vi "Cool vision code.vi"(11 "Image":T1) -> (1 "Original Image":T1(plugin-control), 2 "Distance (ft)":dbl, 3 "Mask":T1(plugin-control))   [LabVIEW 2019]
uses:
  Support/Camera Types.ctl
  <vilib>/vision/Image Controls.llb/IMAQ Image.ctl
  <vilib>/vision/NI_Vision_Development_Module.lvlib
panel:
  out "Disqualified":i32=13
  out "Results":T2(array[cluster])=[{"diameter points"={"first point"={"x"=213.0, "y"=163.0}, "projected point"={"x"=293.0, "y"=194.0}}, "Normalized Center"={"x"=0.58125, "y"=0.48750000000000004}, "Overall Score"=61.175669724085026, "Area Score"=96.13589211618256, "Moment Score"=62.73202614698161, "Aspect Score"=24.659090909090907, "Distance (ft)"=4.347709612348454, "Upper Goal"=FALSE}, {"diameter points"={"first point"={"x"=243.0, "y"=142.0}, "projected point"={"x"=266.0, "y"=171.0}}, "Normalized Center"={"x"=0.5906250000000002, "y"=0.3041666666666667}, "Overall Score"=74.56623386292142, "Area Score"=82.18546637744035, "Moment Score"=61.2760810611263, "Aspect Score"=80.23715415019763, "Distance (ft)"=15.122468216864188, "Upper Goal"=FALSE}] {"Normalized Center"."x" format="%#_2g"; "Normalized Center"."y" format="%#_2g"; "Overall Score" format="%#_2g"; "Distance (ft)" format="%#_3g"; "Area Score" format="%#_2g"; "Moment Score" format="%#_2g"; "Aspect Score" format="%#_2g"}
  in  "Size Limit %":dbl=0.04 min=0.0 max=100.0 step=0.01 format="%#_13g"
  in  "Color Mode":u16(ring)=2 items=["RGB", "HSL", "HSV", "HSI"]
  in  "Particle Count":i32=5
  in  "Score Threshold %":dbl=75.0
  in  "Std Devs for Calibration":cluster{"H":dbl, "S":dbl, "V":dbl}={"H"=4.0, "S"=8.0, "V"=8.0}
  in  "Camera Type (for distance)":T3=enum."MS HD3000 square"
  in  "Annotate":bool=TRUE
  out "Qualified":i32=5
  in  "LED Color Range":T4={"Hue"={14.360681298918061, 47.91090746924753}, "Sat"={75.89285714285714, 255.0}, "Val"={97.14285714285714, 251.32874298095703}} {"Hue" scale=0.0..255.0 scale format="%#_3g"}
  # "Limits"
  # "Particle Results"
  # "Good target"
  # "Disqualified"
  # "Distance (ft)"
  # "Scores"
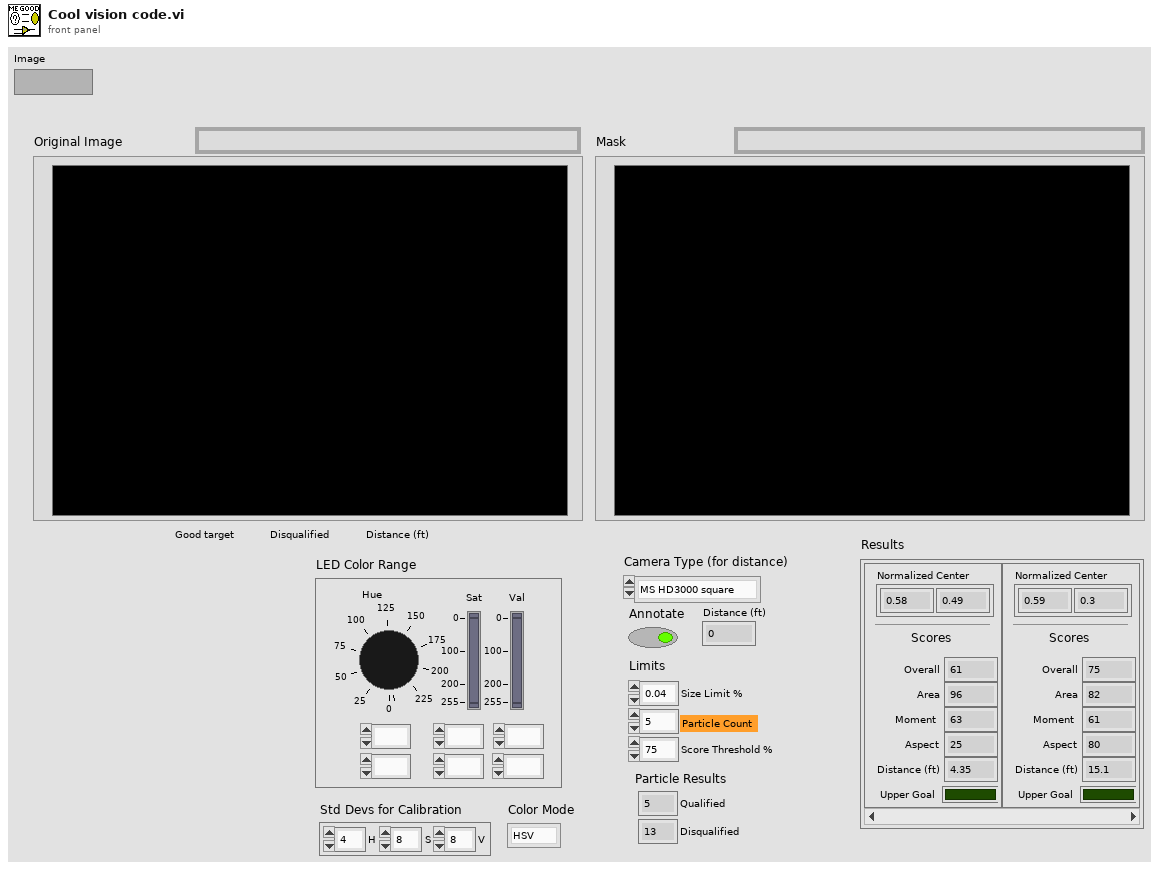
[diagram p1: front panel]
types:
  T1 = typedef "IMAQ Image.ctl" = refnum<image>
  T2 = cluster{"diameter points":cluster{"first point":cluster{"x":dbl, "y":dbl}, "projected point":cluster{"x":dbl, "y":dbl}}, "Normalized Center":cluster{"x":dbl, "y":dbl}, "Overall Score":dbl, "Area Score":dbl, "Moment Score":dbl, "Aspect Score":dbl, "Distance (ft)":dbl, "Upper Goal":bool}[]
  T3 = typedef "Camera Types.ctl" = enum16{"206", "1011", "1013", "MS HD3000 square", "MS HD3000 640x480"}
  T4 = cluster{"Hue":cluster{dbl, dbl}, "Sat":cluster{dbl, dbl}, "Val":cluster{dbl, dbl}}
  T5 = typedef "Particle Parameters" = i32
  T6 = typedef "Image Type" = u32
  T7 = enum32{"AutoM", "Close", "Dilate", "Erode", "Gradient", "Gradient out", "Gradient in", "Hit miss", "Open", "PClose", "POpen", "Thick", "Thin"}
  T8 = cluster{cluster{dbl, dbl}, cluster{dbl, dbl}, cluster{dbl, dbl}}
  T9 = cluster{"remainder":i32, "size":bool, "count":bool}
  T10 = typedef "Target Fields.ctl" = cluster{"diameter points":cluster{"first point":cluster{"x":dbl, "y":dbl}, "projected point":cluster{"x":dbl, "y":dbl}}, "normalized center":cluster{"x":dbl, "y":dbl}, "Overall Score":dbl, "Area Score":dbl, "Moment Score":dbl, "Aspect Score":dbl, "Distance (ft)":dbl, "Upper Goal":bool}
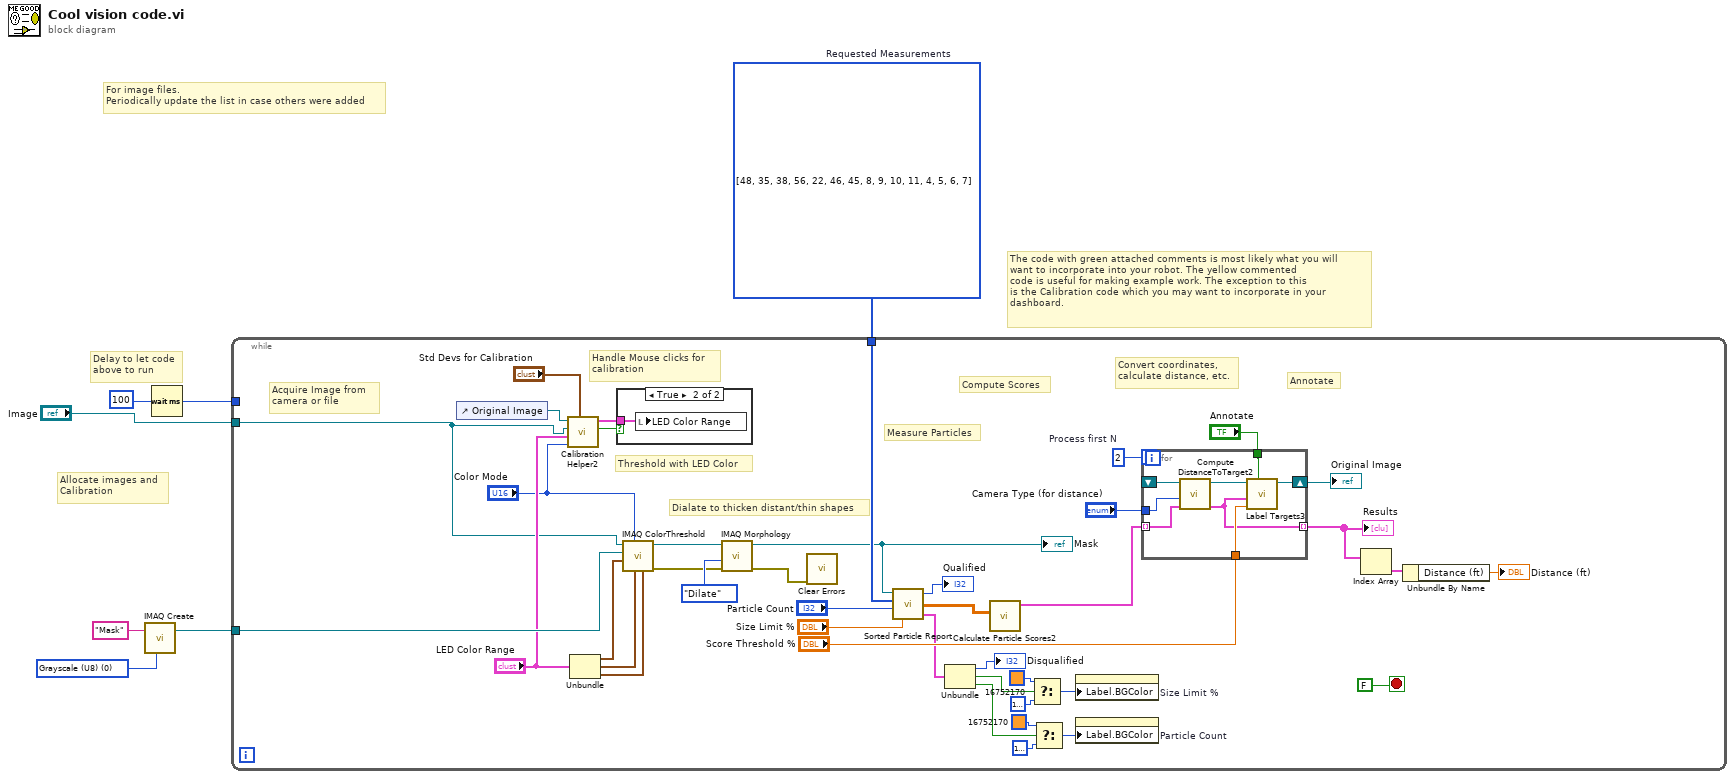
[diagram p0: block diagram]
diagram:
  w4 = T5[] [48, 35, 38, 56, 22, 46, 45, 8, 9, 10, 11, 4, 5, 6, 7] items=["Center of Mass X", "Center of Mass Y", "First Pixel X", "First Pixel Y", "Bounding Rect Left", "Bounding Rect Top", "Bounding Rect Right", "Bounding Rect Bottom", "Max Feret Diameter Start X", "Max Feret Diameter Start Y", "Max Feret Diameter End X", "Max Feret Diameter End Y", "Max Horiz. Segment Length Left", "Max Horiz. Segment Length Right", "Max Horiz. Segment Length Row", "-", "Bounding Rect Width", "Bounding Rect Height", "Bounding Rect Diagonal", "Perimeter", "Convex Hull Perimeter", "Holes' Perimeter", "Max Feret Diameter", "Equivalent Ellipse Major Axis", "Equivalent Ellipse Minor Axis", "Equivalent Ellipse Minor Axis (Feret)", "Equivalent Rect Long Side", "Equivalent Rect Short Side", "Equivalent Rect Diagonal", "Equivalent Rect Short Side (Feret)", "Average Horiz. Segment Length", "Average Vert. Segment Length", "Hydraulic Radius", "Waddel Disk Diameter", "-", "Area", "Holes' Area", "Particle & Holes' Area", "Convex Hull Area", "Image Area", "-", "Number of Holes", "Number of Horiz. Segments", "Number of Vert. Segments", "-", "Orientation", "Max Feret Diameter Orientation", "-", "% Area/Image Area", "% Area/(Particle & Holes' Area)", "Ratio of Equivalent Ellipse Axes", "Ratio of Equivalent Rect Sides", "-", "Elongation Factor", "Compactness Factor", "Heywood Circularity Factor", "Type Factor", "-", "Sum X", "Sum Y", "Sum XX", "Sum XY", "Sum YY", "Sum XXX", "Sum XXY", "Sum XYY", "Sum YYY", "-", "Moment of Inertia XX", "Moment of Inertia XY", "Moment of Inertia YY", "Moment of Inertia XXX", "Moment of Inertia XXY", "Moment of Inertia XYY", "Moment of Inertia YYY", "Norm. Moment of Inertia XX", "Norm. Moment of Inertia XY", "Norm. Moment of Inertia YY", "Norm. Moment of Inertia XXX", "Norm. Moment of Inertia XXY", "Norm. Moment of Inertia XYY", "Norm. Moment of Inertia YYY", "Hu Moment 1", "Hu Moment 2", "Hu Moment 3", "Hu Moment 4", "Hu Moment 5", "Hu Moment 6", "Hu Moment 7"]  # Requested Measurements
  w7 = T6 0 items=["Grayscale (U8)", "Grayscale (I16)", "Grayscale (SGL)", "Complex (CSG)", "RGB (U32)", "HSL (U32)", "RGB (U64)", "Grayscale (U16)"] ("Image Type")
  # "Delay to let code\nabove to run"
  # "The code with green attached comments is most likely what you will\nwant to incorporate into your robot. The yellow commented\ncode is useful for making example work. The exception to this\nis the Calibration code which you may want to incorporate in your\ndashboard."
  # "For image files.\nPeriodically update the list in case others were added"
  # "Allocate images and\nCalibration"
  n1 = call "IMAQ Create"("Image Name"="Mask", "Image Type"=w7) -> ("New Image"=w5:T1)  [unwired: 2 in, 2 out]
  n2 = Wait (ms)(milliseconds to wait=u32 100) -> (millisecond timer value=w3:u32)
  n3 = while {
    tunnel: w5 -> [w47]
    tunnel: w4 -> [w43]
    tunnel: w3 -> [_]
    tunnel: "Image" -> [w11]
    stop <- FALSE stop-if-true
    w30 = 2  # Process first N
    # "Dialate to thicken distant/thin shapes"
    # "Handle Mouse clicks for\ncalibration"
    # "Measure Particles"
    # "Convert coordinates,\ncalculate distance, etc."
    # "Annotate"
    # "Compute Scores"
    # "Threshold with LED Color"
    # "Acquire Image from\ncamera or file"
    n4 = control-ref of="Original Image"() -> (w40:refnum<vi>)
    n5 = call "Calibration Helper2.vi"("Std Devs"="Std Devs for Calibration", "Color Mode"="Color Mode", "Color Components"="LED Color Range", "Image"=w11, "Image Ctl Refnum"=w40) -> ("Changed"=w39:bool, "output color"=w38:T8)  [unwired: 5 in]
    n6 = Unbundle("LED Color Range") -> ("Hue"=w46:cluster{dbl, dbl}, "Sat"=w45:cluster{dbl, dbl}, "Val"=w44:cluster{dbl, dbl})
    n7 = case shown="True" w39 {
      tunnel: w38 -> [_ w57]
      frame False {
      }
      frame True {
        n8 = local write "LED Color Range"(w57) -> ()
      }
    }
    n9 = call "IMAQ ColorThreshold"("Blue or Luma or Val or Inten Range"=w44, "Green or Sat Range"=w45, "Color Mode"="Color Mode", "Red or Hue Range"=w46, "Image Dst"=w47, "Image Src"=w11) -> ("error out"=w27:errorcluster, "Image Dst Out"=w29:T1)  [unwired: 4 in]
    n10 = call "IMAQ Morphology"("error in (no error)"=w27, "Operation"=T7."Dilate", "Image Src"=w29) -> ("error out"=w26:errorcluster, "Image Dst Out"=w23:T1)  [unwired: 7 in]
    "Mask" <- w23
    n11 = call <vilib>:"Clear Errors.vi"("error in (no error)"=w26) -> ()  [unwired: 5 in, 2 out]
    n12 = call "Sorted Particle Report.vi"("Min Area Size %"="Size Limit %", "Particle Count Limit"="Particle Count", "Pixel Measurements"=w43, "Image in"=w23) -> ("limits"=w21:T9, "Sorted Data"=w25:dbl[][], "Particles"=→"Qualified":i32)
    n13 = Unbundle(w21) -> ("remainder"=→"Disqualified":i32, "size"=w15:bool, "count"=w14:bool)
    n14 = call "Calculate Particle Scores2.vi"("Sorted Data"=w25) -> ("Scores"=w24:T10[])  [unwired: 10 in]
    n15 = Select(t=u32 16752170 ("Color"), s=w15, f=u32 16777216 ("Color")) -> (s? t:f=w13:u32)
    n16 = Select(t=u32 16752170 ("Color"), s=w14, f=u32 16777216 ("Color")) -> (s? t:f=w12:u32)
    n17 = property on="Size Limit %" class="DigNum (strict)"("Label.BGColor"=w13) -> ()  [unwired: 2 in, 2 out]
    n18 = property on="Particle Count" class="DigNum (strict)"("Label.BGColor"=w12) -> ()  [unwired: 2 in, 2 out]
    n19 = for {
      N: w30 -> [_]
      tunnel: w24 -> [w54] mode=indexing
      tunnel: "Camera Type (for distance)" -> [w56]
      tunnel: "Annotate" -> [w51]
      shift-right: [w55] -> w31
      shift-left: _ -> [w53]
      tunnel: "Score Threshold %" -> [w50]
      tunnel: [w49] -> w10 mode=indexing
      n20 = call "Compute DistanceToTarget2.vi"("results"=w54, "Camera Type"=w56, "Image Src"=w53) -> ("results out"=w49:T10, "Image Dst Out"=w52:T1)  [unwired: 7 in]
      n21 = call "Label Targets3.vi"("Annotate"=w51, "Score Threshold"=w50, "results"=w49, "Image in"=w52) -> ("Image out"=w55:T1)  [unwired: 7 in]
    }
    "Original Image" <- w31
    "Results" <- w10
    n22 = Index Array(array=w10) -> (element=w9:T10)  [unwired: 1 in]
    n23 = Unbundle By Name(w9) -> ("Distance (ft)"=→"Distance (ft)":dbl)
  }
